vi "get_speed_params.vi"(8 "error in (no error)":errorcluster, 11 "ImagingModeDL090130Frame in":refnum<class "ImagingModeDL090130Frame.lvclass">) -> (0 "error out":errorcluster, 1 "line-scan time":dbl[unit], 2 "frame rate":dbl[unit], 3 "ImagingModeDL090130Frame out":refnum<class "ImagingModeDL090130Frame.lvclass">, 4 "pixel dwell time":dbl[unit], 5 "which one is correct for sure?":T1)   [LabVIEW 2010, in "ImagingModeDL090130Frame.lvclass"]
uses:
  ImagingModeDL090130Frame.lvclass
  speed_parameter_cluster.ctl
  ImagingModeDL090130Frame.lvclass/ImagingModeDL090130Frame.ctl
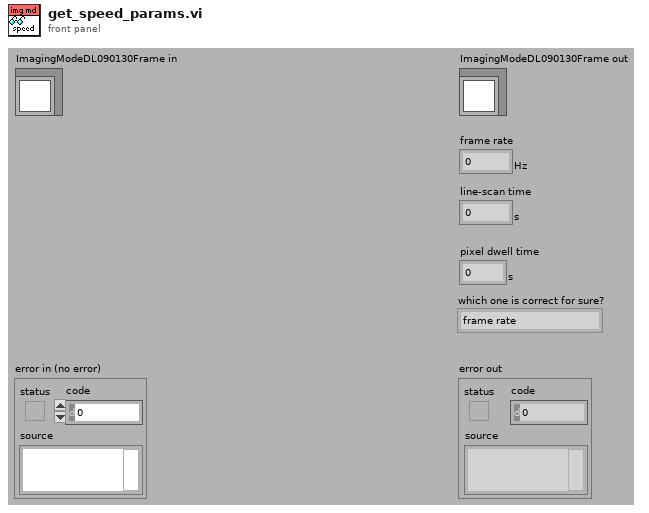
[diagram p1: front panel]
types:
  T1 = typedef "ImagingModeDL090130Frame.lvclass/speed_parameter_cluster.ctl" = enum16{"frame rate", "line-scan time", "pixel-dwell time"}
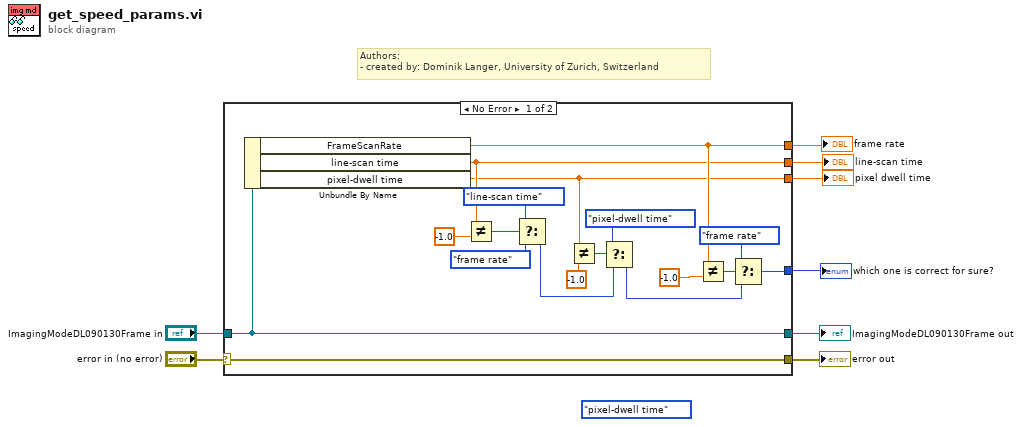
[diagram p0: block diagram]
diagram:
  (unwired) speed_parameter_cluster."pixel-dwell time" ("what changed?")
  # "Authors: \n- created by: Dominik Langer, University of Zurich, Switzerland"
  n1 = case shown="No Error" "error in (no error)" {
    selector: "error in (no error)" -> [w25 w28]
    tunnel: [w25 w28] -> w7
    tunnel: [w26 w27] -> w5
    tunnel: "ImagingModeDL090130Frame in" -> [w26 w27]
    tunnel: [w24 _] -> w4
    tunnel: [w22 _] -> w3
    tunnel: [w21 _] -> w2
    tunnel: [w13 _] -> w1
    frame No Error {
      n2 = Unbundle By Name(w26) -> ("FrameScanRate"=w24:dbl[unit], "line-scan time"=w22:dbl[unit], "pixel-dwell time"=w21:dbl[unit])
      n3 = Not Equal?(x=w22, y=dbl[unit] -1.0) -> (x != y?=w18:bool)
      n4 = Select(t=speed_parameter_cluster."line-scan time" ("what changed?"), s=w18, f=speed_parameter_cluster."frame rate" ("what changed?")) -> (s? t:f=w10:T1)
      n5 = Not Equal?(x=w21, y=dbl[unit] -1.0) -> (x != y?=w15:bool)
      n6 = Select(t=speed_parameter_cluster."pixel-dwell time" ("what changed?"), s=w15, f=w10) -> (s? t:f=w9:T1)
      n7 = Not Equal?(x=w24, y=dbl[unit] -1.0) -> (x != y?=w14:bool)
      n8 = Select(t=speed_parameter_cluster."frame rate" ("what changed?"), s=w14, f=w9) -> (s? t:f=w13:T1)
    }
    frame Error {
    }
  }
  "error out" <- w7
  "ImagingModeDL090130Frame out" <- w5
  "frame rate" <- w4
  "line-scan time" <- w3
  "pixel dwell time" <- w2
  "which one is correct for sure?" <- w1
